vi "test - Build Evaluation String - I32_EW.vi"(8 "error in (no error)":errorcluster, 11 "TestCase in":refnum<class "Create New Assert Tester.lvclass">) -> (0 "error out":errorcluster, 3 "TestCase out":refnum<class "Create New Assert Tester.lvclass">)   [LabVIEW 2017, in "Create New Assert Tester.lvclass"]
uses:
  Create New Assert Tester.lvclass
  <vilib>/Utility/Data Type/Type Definitions/Data Type.ctl
  <vilib>/addons/_JKI Toolkits/VI Tester/TestCase.llb/TestCase.lvclass
  <vilib>/Utility/Data Type/NI_Data Type.lvlib
  C:/Program Files (x86)/National Instruments/LabVIEW 2017/vi.lib/addons/_JKI Toolkits/VI Tester/TestCase.llb/TestCase.lvclass
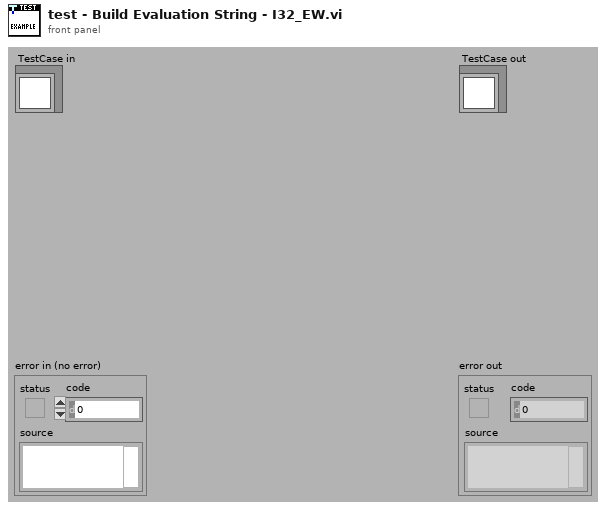
[diagram p1: front panel]
types:
  T1 = typedef "NI_Data Type.lvlib/Data Type.ctl" = enum8{"Invalid Type", "Void", "I8", "I16", "I32", "I64", "U8", "U16", "U32", "U64", "Single Float", "Double Float", "Extended Float", "Single Complex", "Double Complex", "Extended Complex", "Enum U8", "Enum U16", "Enum U32", "Enum U64", "Single Float With Unit", "Double Float With Unit", "Extended Float With Unit", "Single Complex with Unit", "Double Complex with Unit", "Extended Complex with Unit", "Boolean", "String", "Path", "Picture", "Tag", "Array", "Cluster", "Variant", "LV Variant", "Waveform", "Timestamp", "Digital Waveform", "Digital Data", "ExpressData", "Refnum", "External Data", "VI", "Poly VI", "LabVIEW Class Instance", "Fixed Point"}
  T2 = typedef "Assert Scripting Configuration.ctl" = cluster{"Assert Name":string, "Comment":string, "Numeric Operation":string, "Type":T1, "String Operation":string, "DBL Comparison Value 1":dbl, "DBL Comparison Value 2":dbl, "I32 Comparison Value 1":i32, "I32 Comparison Value 2":i32, "Creator":string, "Creation Timestamp":timestamp, "String Comparison Value":string, "Description":string, "Default Failure Action":enum16{"None", "Log To File", "Pause Execution", "Abort Execution"}, "Boolean Comparison Value":bool, "I8 Comparison Value 1":i8, "I8 Comparison Value 2":i8, "I16 Comparison Value 1":i16, "I16 Comparison Value 2":i16, "I64 Comparison Value 1":i64, "I64 Comparison Value 2":i64, "U8 Comparison Value 1":u8, "U8 Comparison Value 2":u8, "U16 Comparison Value 1":u16, "U16 Comparison Value 2":u16, "U32 Comparison Value 1":u32, "U32 Comparison Value 2":u32, "U64 Comparison Value 1":u64, "U64 Comparison Value 2":u64, "EXT Comparison Value 1":ext, "EXT Comparison Value 2":ext, "SGL Comparison Value 1":sgl, "SGL Comparison Value 2":sgl, "Float Digits of Precision":u8}
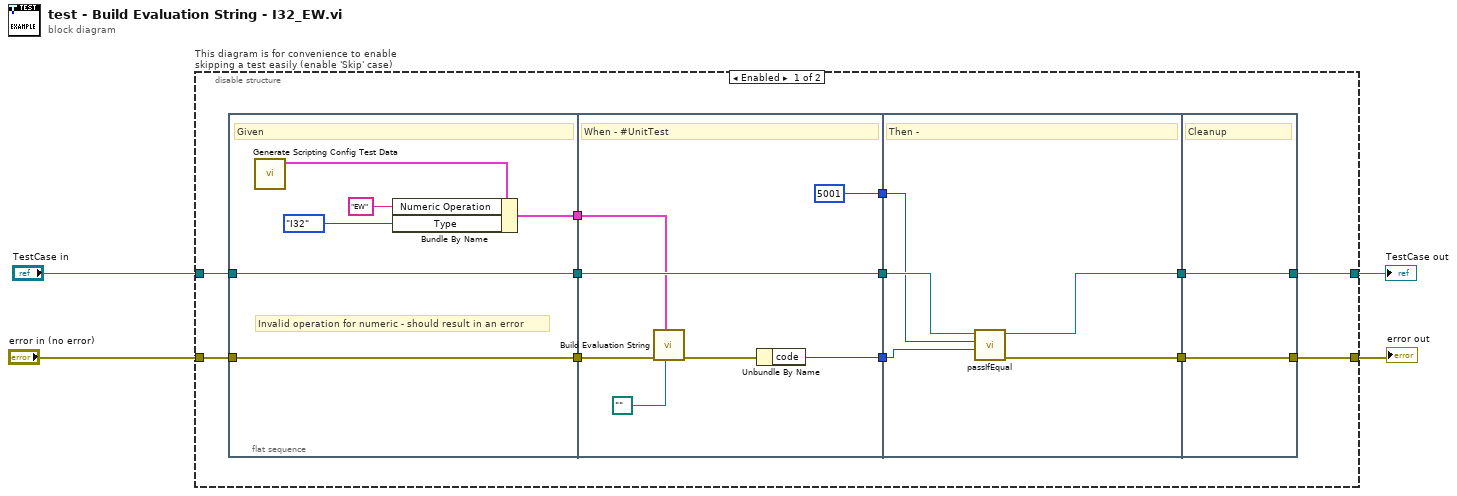
[diagram p0: block diagram]
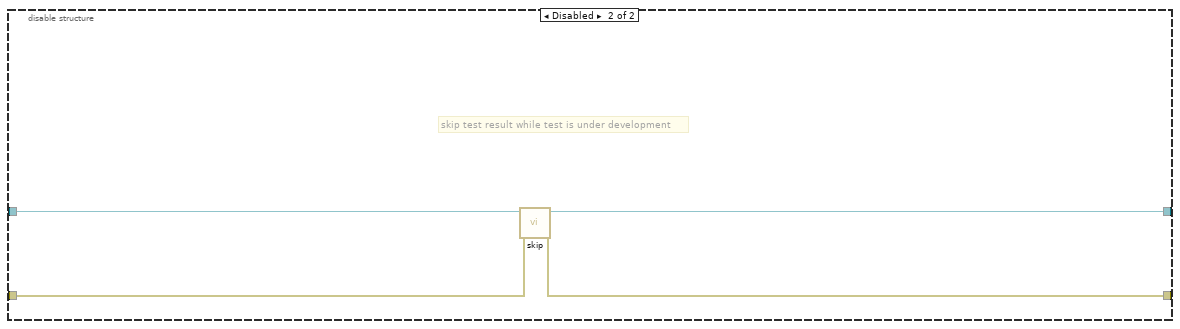
[diagram p2: hidden frame]
diagram:
  n1 = disable-structure "This diagram is for convenience to enable skipping a test easily (enable 'Skip' case)" shown="Enabled" {
    disable-tunnel: "TestCase in" -> [w10 w40]
    disable-tunnel: [w7 w38] -> w1
    disable-tunnel: [w8 w39] -> w3
    disable-tunnel: "error in (no error)" -> [w9 w37]
    frame Enabled {
      n2 = flat-sequence {
        tunnel: w9 -> [w17]
        tunnel: w10 -> [w22]
        tunnel: [w22] -> w16
        tunnel: [w17] -> w15
        tunnel: [w18] -> w6
        tunnel: [w29] -> w14
        tunnel: [w23] -> w13
        tunnel: w16 -> [w29]
        tunnel: w15 -> [w28]
        tunnel: w6 -> [w26]
        tunnel: [5001] -> w5
        tunnel: [w32] -> w12
        tunnel: [w34] -> w11
        tunnel: w14 -> [w33]
        tunnel: w13 -> [w31]
        tunnel: w5 -> [w30]
        tunnel: [w35] -> w8
        tunnel: [w36] -> w7
        tunnel: w12 -> [w36]
        tunnel: w11 -> [w35]
        frame #0 {
          # "Invalid operation for numeric - should result in an error"
          # "Given"
          n3 = call "Generate Scripting Config Test Data.vi"() -> ("Assert Scripting Configuration"=w21:T2)  [unwired: 11 in]
          n4 = Bundle By Name(cluster=w21, "Numeric Operation"="EW", "Type"=Data_Type."I32") -> (w18:T2)
        }
        frame #1 {
          # "When - #UnitTest"
          n5 = call "Build Evaluation String.vi"("VI Path"=path "", "Assert Scripting Configuration"=w26, "error in (no error)"=w28) -> ("error out"=w27:errorcluster)  [unwired: 7 in, 1 out]
          n6 = Unbundle By Name(w27) -> ("code"=w23:i32)
        }
        frame #2 {
          # "Then -"
          n7 = call-dynamic "passIfEqual.vi"("y"=w31, "x"=w30, "TestCase in"=w33) -> ("error out"=w34:errorcluster, "TestCase out"=w32:refnum<class "Create New Assert Tester.lvclass">)  [unwired: 7 in]
        }
        frame #3 {
          # "Cleanup"
        }
      }
    }
    frame Disabled {
      # "skip test result while test is under development"
      n8 = call <vilib>:"skip.vi"("error in (no error)"=w37, "TestCase in"=w40) -> ("error out"=w39:errorcluster, "TestCase out"=w38:refnum<class "Create New Assert Tester.lvclass">)  [unwired: 8 in]
    }
  }
  "error out" <- w3
  "TestCase out" <- w1
